vi "DMA.Write (Scatter-Gather).vi"(7 "timeout ms (1000)":u32=1000, 8 "error in (no error)":errorcluster, 10 "Scatter-Gather Transfer Spec":T1 {"Block Descriptors"."next descriptor ptr" format="%08x"; "Block Descriptors"."data size" format="%08x"; "Block Descriptors"."data ptr (upper)" format="%08x"; "Block Descriptors"."data ptr (lower)" format="%08x"; "Block Descriptors"."descriptor ptr (aligned)" format="%08x"; "Block Descriptors"."descriptor size" format="%08x"; "Block Descriptors"."descriptor ptr (VISA)" format="%08x"; "RFM Address" format="%08x"}, 11 "GE 5565PIORC":refnum<class "GE 5565PIORC.lvclass">) -> (0 "error out":errorcluster, 1 "Timed out?":bool, 3 "GE 5565PIORC out":refnum<class "GE 5565PIORC.lvclass">)   [LabVIEW 2016, in "GE 5565PIORC.lvclass"]
uses:
  GE 5565PIORC.lvclass
  Controls/DMA Transfer Spec (Scatter-Gather).ctl
  Controls/DMA Block Descriptor.ctl
  GE 5565PIORC.lvclass/GE 5565PIORC.ctl
  DMA.Configure (Scatter-Gather).vi
  Registers/Local Configuration.DMAMODE0.Scatter-Gather Enable.Set.vi
  Registers/Local Configuration.Local Address.Set.vi
  Registers/Local Configuration.Transfer Size.Set.vi
  Registers/Local Configuration.DMADPR0.First Descriptor Address.Set.vi
  Registers/Local Configuration.DMADPR0.Transfer Direction.Set.vi
  Registers/Local Configuration.DMACSR0.DMA Start.Set.vi
  Interrupts/Wait for PXI Interrupt Events.vi
  Registers/Local Configuration.DMACSR0.DMA Clear Interrupt.Set.vi
  <vilib>/Utility/error.llb/Clear Errors.vi
  Binary Operations/Set Bits.vi
  Binary Operations/Set Bits U32.vi
  Registers/Local Configuration.Get Register Offset.vi
  Binary Operations/Get Bits.vi
  Binary Operations/Get Bits U32.vi
  Scatter-Gather/DMA.Scatter-Gather.Get Transfer Size.vi
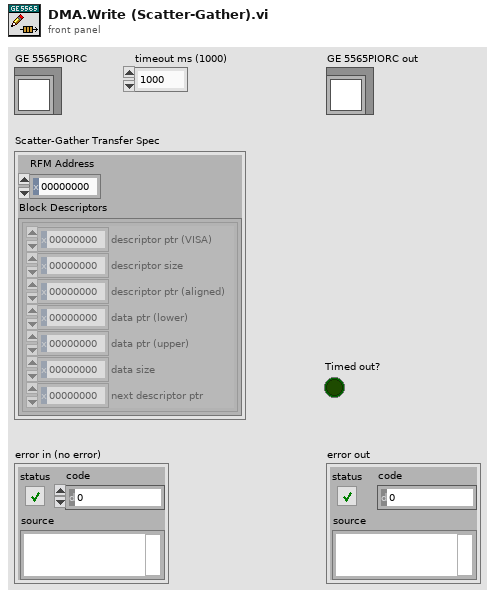
[diagram p1: front panel]
types:
  T1 = typedef "GE 5565PIORC.lvclass/DMA Transfer Spec (Scatter-Gather).ctl" = cluster{"RFM Address":u32, "Block Descriptors":T2[]}
  T2 = typedef "GE 5565PIORC.lvclass/DMA Block Descriptor.ctl" = cluster{"descriptor ptr (VISA)":u32, "descriptor size":u32, "descriptor ptr (aligned)":u32, "data ptr (lower)":u32, "data ptr (upper)":u32, "data size":u32, "next descriptor ptr":u32}
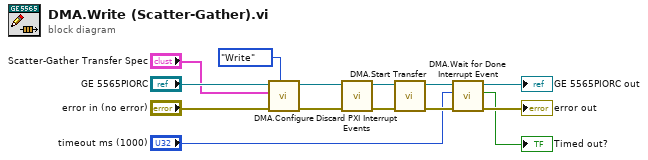
[diagram p0: block diagram]
diagram:
  n1 = call-poly "DMA.Configure.vi"("Transfer Direction"=enum16{"Write", "Read"}."Write", "error in (no error)"="error in (no error)", "Scatter-Gather Transfer Spec"="Scatter-Gather Transfer Spec", "GE 5565PIORC"="GE 5565PIORC") -> ("error out"=w4:errorcluster, "GE 5565PIORC out"=w3:refnum<class "GE 5565PIORC.lvclass">)  [unwired: 6 in]
  n2 = call "Discard PXI Interrupt Events.vi"("error in (no error)"=w4, "GE 5565PIORC in"=w3) -> ("error out"=w5:errorcluster, "GE 5565PIORC out"=w6:refnum<class "GE 5565PIORC.lvclass">)  [unwired: 8 in]
  n3 = call "DMA.Start Transfer.vi"("error in (no error)"=w5, "GE 5565PIORC"=w6) -> ("error out"=w10:errorcluster, "GE 5565PIORC out"=w11:refnum<class "GE 5565PIORC.lvclass">)  [unwired: 8 in]
  n4 = call "DMA.Wait for Done Interrupt Event.vi"("error in (no error)"=w10, "timeout ms (1000)"="timeout ms (1000)", "GE 5565PIORC"=w11) -> ("error out"=→"error out":errorcluster, "Timed out?"=→"Timed out?":bool, "GE 5565PIORC out"=→"GE 5565PIORC out":refnum<class "GE 5565PIORC.lvclass">)  [unwired: 6 in]
